vi "configAO_function.vi"(5 "Port":u16, 7 "address":string, 8 "error in (no error)":errorcluster, 9 "Function":T1, 10 "AO Channel":T2 min=1 max=16, 11 "Instrument.Lockin in":refnum<class "Instrument.Lockin.lvclass">) -> (0 "error out":errorcluster, 3 "Instrument.Lockin out":refnum<class "Instrument.Lockin.lvclass">)   [LabVIEW 2016]
doc: "API to configure an AO function.\n\nSpecify which channel you want to change and the value you want to set.\n\nIf address=\"\", this API reads from localhost\nIf address is remote lockin, you need to add this computer to allowed whitelist on the lockin computer you are trying to access."
uses:
  Instrument.Lockin/Typedefs/AO_Channel-Numeric.ctl
  Instrument.Lockin/Typedefs/Function-enum.ctl
  Instrument.Lockin/Instrument.Lockin.lvclass
  Instrument.Lockin/Typedefs/Instrument.Lockin.Commands--Enum.ctl
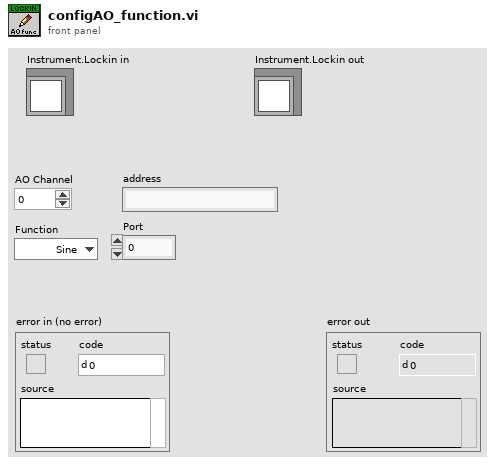
[diagram p1: front panel]
types:
  T1 = typedef "Instrument.Lockin.lvclass/Function-enum.ctl" = enum16{"Sine", "Triangle", "Square", "Sawtooth"}
  T2 = typedef "Instrument.Lockin.lvclass/AO_Channel-Numeric.ctl" = i32
  T3 = typedef "Instrument.Lockin.lvclass/Instrument.Lockin.Commands--Enum.ctl" = enum16{"configAO", "configAO_Amplitude", "configAO_DC", "configAO_Frequency", "configAO_Phase", "configAO_Function", "configAO_I+", "configREF", "configREF_Frequency", "configREF_Phase", "configREF_Filter", "configIVmode", "Reset", "configSampling", "Trigger", "getAO", "getAI", "getResults", "getTrigger", "getIVmode", "getSampling", "getAOconfig", "getREFconfig", "getREF_Filter", "configGain", "getGain", "configAutoSampling", "getAutoSampling"}
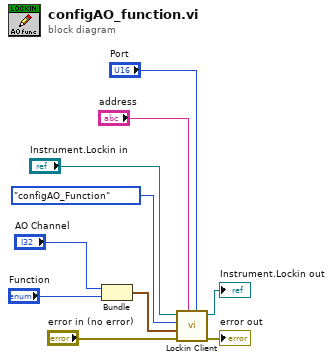
[diagram p0: block diagram]
diagram:
  n1 = Bundle("AO Channel"="AO Channel", "Function"="Function") -> (w10:cluster{"AO Channel":T2, "Function":T1})  [unwired: 1 in]
  n2 = call "Lockin Client.vi"("Port"="Port", "address"="address", "error in (no error)"="error in (no error)", "Data"=w10, "Command"=Instrument.Lockin.Commands--Enum."configAO_Function", "Instrument.Lockin in"="Instrument.Lockin in") -> ("error out"=→"error out":errorcluster, "Instrument.Lockin out"=→"Instrument.Lockin out":refnum<class "Instrument.Lockin.lvclass">)  [unwired: 3 in, 1 out]
